vi "参数初始化.vi"   [LabVIEW 2016]
types:
  T1 = typedef "数据库类型.ctl" = enum16{"Access", "SQLite"}
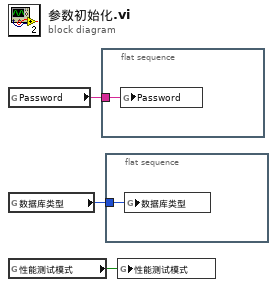
[diagram p0: block diagram]
diagram:
  n1 = global read "非断电保持全局变量.vi" "Password"() -> (w1:string)
  n2 = global read "非断电保持全局变量.vi" "数据库类型"() -> (w2:T1)
  n3 = global read "系统设置全局变量.vi" "性能测试模式"() -> (w3:bool)
  n4 = flat-sequence {
    tunnel: w1 -> [w4]
    frame #0 {
      n5 = global write "外部调用接口全局变量.vi" "Password"(w4) -> ()
    }
  }
  n6 = flat-sequence {
    tunnel: w2 -> [w5]
    frame #0 {
      n7 = global write "外部调用接口全局变量.vi" "数据库类型"(w5) -> ()
    }
  }
  n8 = global write "外部调用接口全局变量.vi" "性能测试模式"(w3) -> ()
